vi "OPCConnection.BuildURL.vi"(10 "Server Port":u16, 11 "Server IP Address":string="localhost") -> (3 "OPC Path":string)   [LabVIEW 2019, in "OPC UA Client Addon Shared.lvlib"]
uses:
  OPC UA Client Addon Shared.lvlib
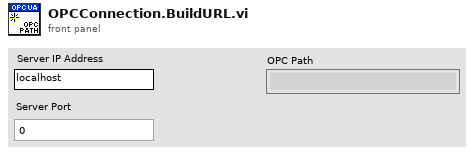
[diagram p1: front panel]
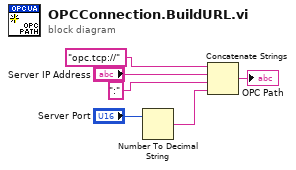
[diagram p0: block diagram]
diagram:
  n1 = Number To Decimal String(number="Server Port") -> (decimal integer string=w4:string)  [unwired: 1 in]
  n2 = Concatenate Strings("opc.tcp://", "Server IP Address", ":", w4) -> (→"OPC Path":string)
